vi "Destroy.vi"(8 "error in (no error)":errorcluster, 11 "ConfigManager.Text in":refnum<class "ConfigManager.Text.lvclass">) -> (0 "error out":errorcluster, 3 "ConfigManager.Text out":refnum<class "ConfigManager.Text.lvclass">)   [LabVIEW 2013, in "CfgManager.Text.lvlib" / "ConfigManager.Text.lvclass"]
uses:
  ConfigManager.Text.lvclass
  ConfigManager.Text.lvclass/ConfigManager.Text.ctl
  <vilib>/Utility/error.llb/Clear Errors.vi
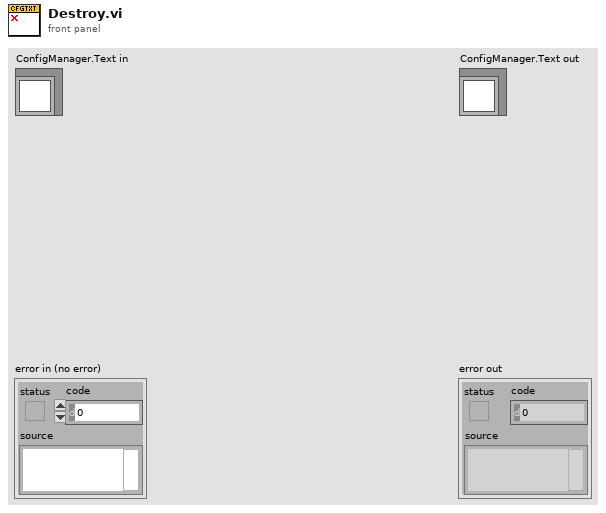
[diagram p1: front panel]
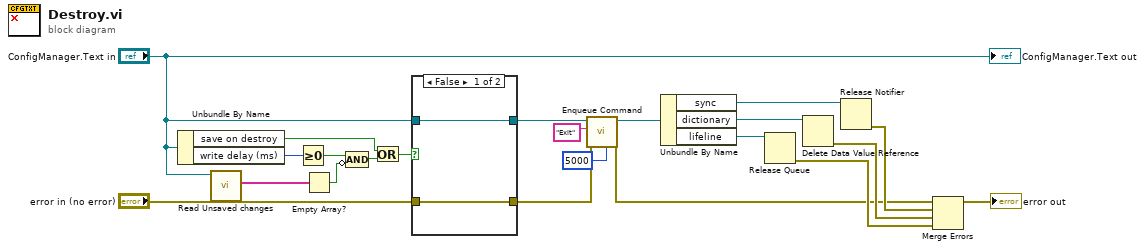
[diagram p0: block diagram]
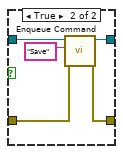
[diagram p2: hidden frame]
diagram:
  n1 = Unbundle By Name("ConfigManager.Text in") -> ("save on destroy"=w5:bool, "write delay (ms)"=w8:i32)
  n2 = call "Read Unsaved changes.vi"("ConfigManager.Text in"="ConfigManager.Text in") -> ("Unsaved changes"=w2:string[])  [unwired: 9 in, 1 out]
  n3 = Greater Or Equal To 0?(x=w8) -> (x >= 0?=w7:bool)
  n4 = Empty Array?(array=w2) -> (empty?=w1:bool)
  n5 = Compound Arithmetic op=AND(w7, invert w1) -> (w6:bool)
  n6 = Or(x=w5, y=w6) -> (x .or. y?=w4:bool)
  n7 = case shown="False" w4 {
    tunnel: "ConfigManager.Text in" -> [w24 w28]
    tunnel: [w24 w27] -> w19
    tunnel: "error in (no error)" -> [w23 w26]
    tunnel: [w23 w25] -> w9
    frame False {
    }
    frame True {
      n8 = call "Enqueue Command.vi"("error in (no error)"=w26, "command"="Save", "ConfigManager.Text in"=w28) -> ("error out"=w25:errorcluster, "ConfigManager.Text out"=w27:refnum<class "ConfigManager.Text.lvclass">)  [unwired: 6 in, 1 out]
    }
  }
  n9 = call "Enqueue Command.vi"("ack timeout (0 ms: no ack)"=5000 ("timeout in ms (-1)"), "error in (no error)"=w9, "command"="Exit", "ConfigManager.Text in"=w19) -> ("error out"=w10:errorcluster, "ConfigManager.Text out"=w18:refnum<class "ConfigManager.Text.lvclass">)  [unwired: 5 in, 1 out]
  n10 = Unbundle By Name(w18) -> ("sync"=w15:refnum<notifier>, "dictionary"=w14:refnum<data-value>, "lifeline"=w13:refnum<queue>)
  n11 = Release Queue(queue=w13) -> (error out=w11:errorcluster)  [unwired: 2 in, 2 out]
  n12 = Delete Data Value Reference(data value reference=w14) -> (error out=w12:errorcluster)  [unwired: 1 in, 1 out]
  n13 = Release Notifier(notifier=w15) -> (error out=w16:errorcluster)  [unwired: 2 in, 2 out]
  n14 = Merge Errors(w10, w16, w12, w11) -> (→"error out":errorcluster)
  "ConfigManager.Text out" <- "ConfigManager.Text in"
